vi "test json to variant path.vi"(8 "error in (no error)":errorcluster) -> (0 "error out":errorcluster)   [LabVIEW 2019, in "labview_json_tests.lvlib"]
uses:
  labview_json_tests.lvlib
  lib/labview_json.lvlib
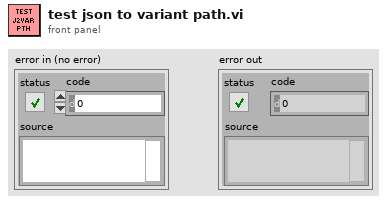
[diagram p1: front panel]
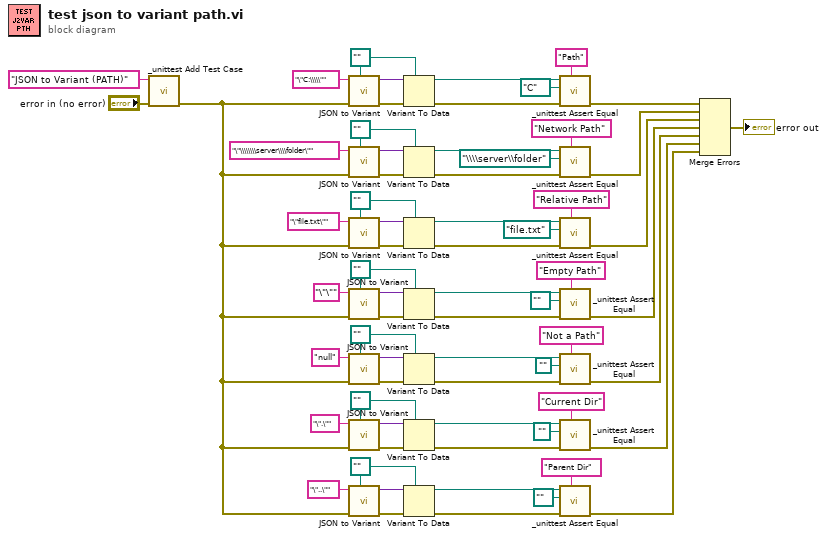
[diagram p0: block diagram]
diagram:
  w10 = path ""
  w16 = path ""
  w28 = path ""
  w31 = path ""
  w34 = path ""
  w38 = path ""
  w40 = path ""
  n1 = call "_unittest Add Test Case.vi"("error in (no error)"="error in (no error)", "Test Case"="JSON to Variant (PATH)") -> ("error out"=w3:errorcluster)  [unwired: 9 in]
  n2 = call "JSON to Variant.vi"("Variant Type"=w40, "error in (no error)"=w3, "JSON"="\"C:\\\\\"") -> ("error out"=w57:errorcluster, "Variant out"=w41:variant)  [unwired: 7 in]
  n3 = call "JSON to Variant.vi"("Variant Type"=w38, "error in (no error)"=w3, "JSON"="\"\\\\\\\\server\\\\folder\"") -> ("error out"=w55:errorcluster, "Variant out"=w42:variant)  [unwired: 7 in]
  n4 = call "JSON to Variant.vi"("Variant Type"=w34, "error in (no error)"=w3, "JSON"="\"file.txt\"") -> ("error out"=w54:errorcluster, "Variant out"=w43:variant)  [unwired: 7 in]
  n5 = call "JSON to Variant.vi"("Variant Type"=w31, "error in (no error)"=w3, "JSON"="\"\"") -> ("error out"=w53:errorcluster, "Variant out"=w44:variant)  [unwired: 7 in]
  n6 = call "JSON to Variant.vi"("Variant Type"=w28, "error in (no error)"=w3, "JSON"="null") -> ("error out"=w24:errorcluster, "Variant out"=w27:variant)  [unwired: 7 in]
  n7 = call "JSON to Variant.vi"("Variant Type"=w16, "error in (no error)"=w3, "JSON"="\".\"") -> ("error out"=w20:errorcluster, "Variant out"=w17:variant)  [unwired: 7 in]
  n8 = call "JSON to Variant.vi"("Variant Type"=w10, "error in (no error)"=w3, "JSON"="\"..\"") -> ("error out"=w6:errorcluster, "Variant out"=w9:variant)  [unwired: 7 in]
  n9 = Variant To Data(error in=w57, type=w40, Variant=w41) -> (data=w39:path, error out=w45:errorcluster)
  n10 = Variant To Data(error in=w55, type=w38, Variant=w42) -> (data=w37:path, error out=w46:errorcluster)
  n11 = Variant To Data(error in=w54, type=w34, Variant=w43) -> (data=w33:path, error out=w47:errorcluster)
  n12 = Variant To Data(error in=w53, type=w31, Variant=w44) -> (data=w30:path, error out=w48:errorcluster)
  n13 = Variant To Data(error in=w24, type=w28, Variant=w27) -> (data=w2:path, error out=w26:errorcluster)
  n14 = Variant To Data(error in=w20, type=w16, Variant=w17) -> (data=w15:path, error out=w18:errorcluster)
  n15 = Variant To Data(error in=w6, type=w10, Variant=w9) -> (data=w11:path, error out=w8:errorcluster)
  n16 = call "_unittest Assert Equal.vi"("Message"="Path", "error in (no error)"=w45, "Expected Value"=path "C:/", "Actual Value"=w39) -> ("error out"=w65:errorcluster)  [unwired: 7 in]
  n17 = call "_unittest Assert Equal.vi"("Message"="Network Path", "error in (no error)"=w46, "Expected Value"=path "\\\\server\\folder", "Actual Value"=w37) -> ("error out"=w62:errorcluster)  [unwired: 7 in]
  n18 = call "_unittest Assert Equal.vi"("Message"="Relative Path", "error in (no error)"=w47, "Expected Value"=path "file.txt", "Actual Value"=w33) -> ("error out"=w59:errorcluster)  [unwired: 7 in]
  n19 = call "_unittest Assert Equal.vi"("Message"="Empty Path", "error in (no error)"=w48, "Expected Value"=path "", "Actual Value"=w30) -> ("error out"=w58:errorcluster)  [unwired: 7 in]
  n20 = call "_unittest Assert Equal.vi"("Message"="Not a Path", "error in (no error)"=w26, "Expected Value"=path "" ("Not A Path Constant"), "Actual Value"=w2) -> ("error out"=w22:errorcluster)  [unwired: 7 in]
  n21 = call "_unittest Assert Equal.vi"("Message"="Current Dir", "error in (no error)"=w18, "Expected Value"=path "", "Actual Value"=w15) -> ("error out"=w13:errorcluster)  [unwired: 7 in]
  n22 = call "_unittest Assert Equal.vi"("Message"="Parent Dir", "error in (no error)"=w8, "Expected Value"=path "..", "Actual Value"=w11) -> ("error out"=w4:errorcluster)  [unwired: 7 in]
  n23 = Merge Errors(w65, w62, w59, w58, w22, w13, w4) -> (→"error out":errorcluster)
